vi "Add_Inlet_Temp_at_Z.vi"() -> (5 "Plug in titles":string[](array[string]), 7 "Plug in values":string[](array[string]))   [LabVIEW 2015]
uses:
  Globals/Meas_global.vi
panel:
  out "Z":dbl
  # "Please enter any run information in the box below"
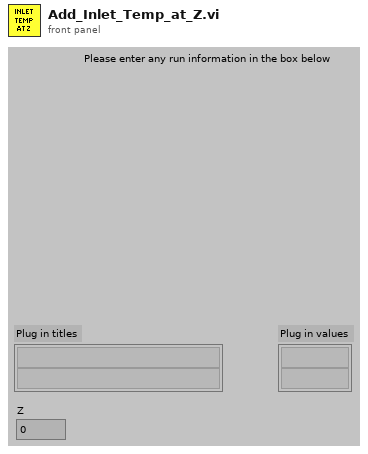
[diagram p1: front panel]
types:
  T1 = typedef "Analysis_info_cluster.ctl" = cluster{"Colour":u32, "Inst type":T2, "Inst name":string, "Symbol":string, "Code name":string, "Extra Info":string, "Inst Array":T3, "Extra Titles":string[], "Extra Values":string[], "U":dbl, "u^2":dbl, "u^3":dbl, "u^4":dbl, "Skew_u":dbl, "Kurt_u":dbl, "Sd Error in Mean":dbl, "% u'/U":dbl, "X":dbl, "Y":dbl, "Z":dbl, "Timescale integral to 25%":dbl, "Sd Error in Variance":dbl, "Calib File":path, "Calib Constants":dbl[], "Output Position":bool, "Full Stats":bool, "Av Sampling Rate":dbl, "Av No of Samples":dbl, "Total Meas Time (s)":dbl, "ADAM Ch Name":string}
  T2 = typedef "Inst_type.ctl" = enum16{"Propeller anemometer", "Raw voltage", "Pressure Transducer", "Pitot-static tube", "Preston tube", "Hot wire", "Cross wire 1", "Cross wire 2", "Generic Linear", "Generic Polynomial", "Generic BackPoly", "Fast FID", "Thermocouple", "Cold wire", "Pulsed Wire", "LDA Vel", "LDA Tran time", "LDA Arr time", "Microphone"}
  T3 = typedef "Instrument_Array.ctl" = enum16{"PWA", "LDA", "Analogue"}
  T4 = typedef "Post_Process.ctl" = enum16{"Take New Data", "Post Process Raw Data File"}
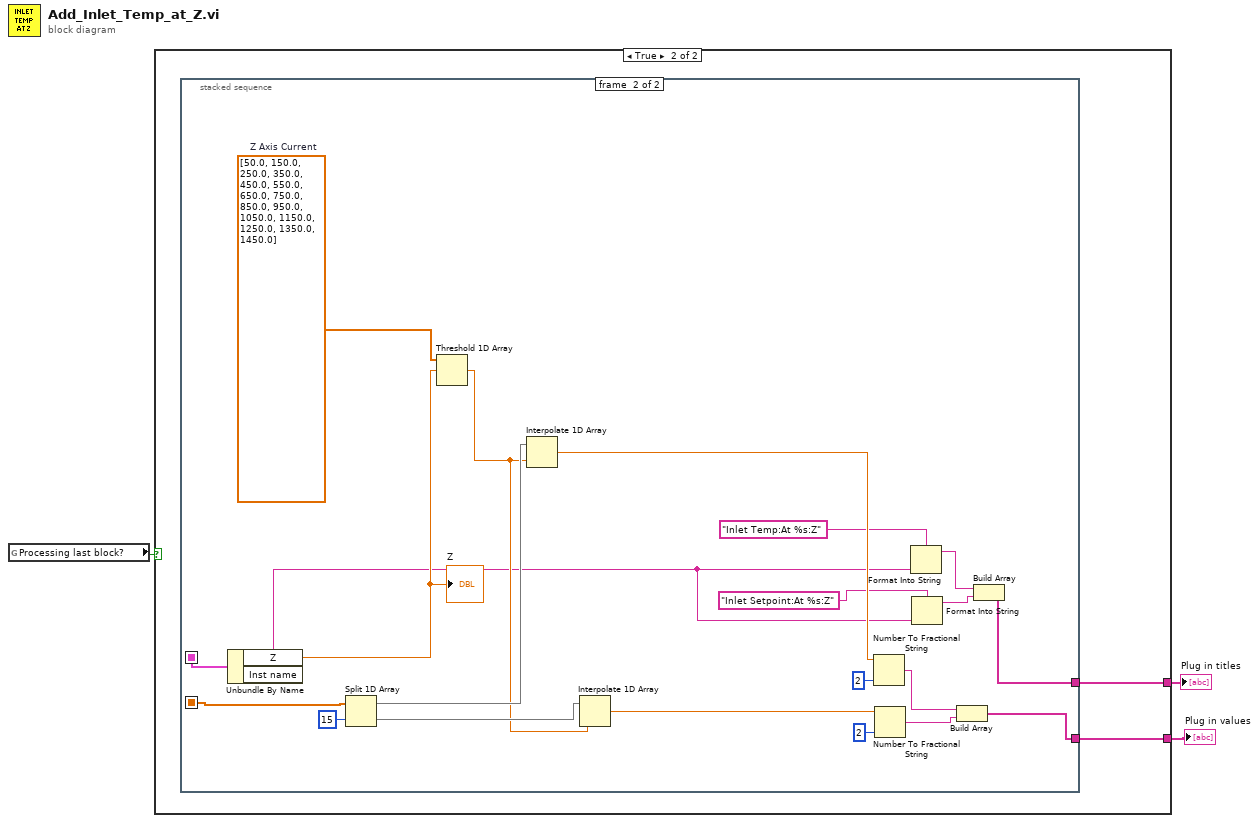
[diagram p0: block diagram]
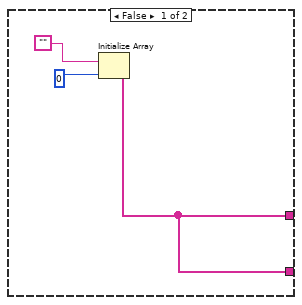
[diagram p2: hidden frame]
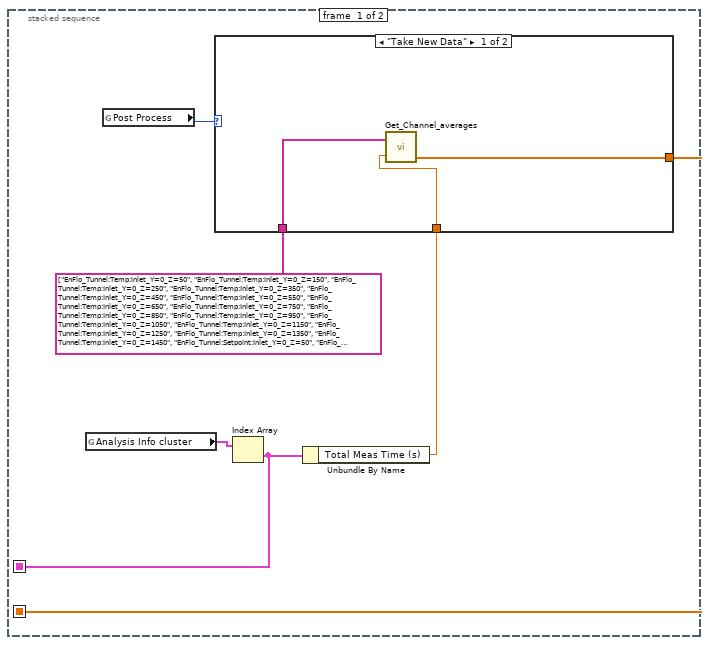
[diagram p3: hidden frame]
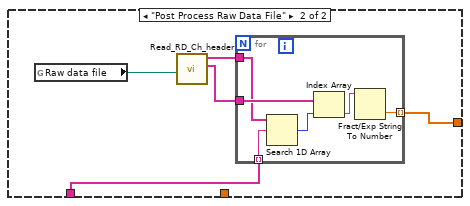
[diagram p4: hidden frame]
diagram:
  n1 = global read "Meas_global.vi" "Processing last block?"() -> (w3:bool)
  n2 = case shown="True" w3 {
    tunnel: [w4 w7] -> w2
    tunnel: [w4 w8] -> w1
    frame False {
      n3 = Initialize Array("", 0) -> (w4:string[])
    }
    frame True {
      n4 = stacked-sequence {
        seq-local: [w11 _] -> [_ w49]
        seq-local: [w9 _] -> [_ w40]
        tunnel: [_ w45] -> w8
        tunnel: [_ w44] -> w7
        frame #0 {
          n5 = global read "Meas_global.vi" "Analysis Info cluster"() -> (w12:T1[])
          n6 = global read "Meas_global.vi" "Post Process"() -> (w14:T4)
          n7 = Index Array(array=w12) -> (element=w11:T1)  [unwired: 1 in]
          n8 = Unbundle By Name(w11) -> ("Total Meas Time (s)"=w10:dbl)
          n9 = case shown="\"Take New Data\"" w14 {
            tunnel: string[] ["EnFlo_Tunnel:Temp:Inlet_Y=0_Z=50", "EnFlo_Tunnel:Temp:Inlet_Y=0_Z=150", "EnFlo_Tunnel:Temp:Inlet_Y=0_Z=250", "EnFlo_Tunnel:Temp:Inlet_Y=0_Z=350", "EnFlo_Tunnel:Temp:Inlet_Y=0_Z=450", "EnFlo_Tunnel:Temp:Inlet_Y=0_Z=550", "EnFlo_Tunnel:Temp:Inlet_Y=0_Z=650", "EnFlo_Tunnel:Temp:Inlet_Y=0_Z=750", "EnFlo_Tunnel:Temp:Inlet_Y=0_Z=850", "EnFlo_Tunnel:Temp:Inlet_Y=0_Z=950", "EnFlo_Tunnel:Temp:Inlet_Y=0_Z=1050", "EnFlo_Tunnel:Temp:Inlet_Y=0_Z=1150", "EnFlo_Tunnel:Temp:Inlet_Y=0_Z=1250", "EnFlo_Tunnel:Temp:Inlet_Y=0_Z=1350", "EnFlo_Tunnel:Temp:Inlet_Y=0_Z=1450", "EnFlo_Tunnel:Setpoint:Inlet_Y=0_Z=50", "EnFlo_Tunnel:Setpoint:Inlet_Y=0_Z=150", "EnFlo_Tunnel:Setpoint:Inlet_Y=0_Z=250", "EnFlo_Tunnel:Setpoint:Inlet_Y=0_Z=350", "EnFlo_Tunnel:Setpoint:Inlet_Y=0_Z=450", "EnFlo_Tunnel:Setpoint:Inlet_Y=0_Z=550", "EnFlo_Tunnel:Setpoint:Inlet_Y=0_Z=650", "EnFlo_Tunnel:Setpoint:Inlet_Y=0_Z=750", "EnFlo_Tunnel:Setpoint:Inlet_Y=0_Z=850", "EnFlo_Tunnel:Setpoint:Inlet_Y=0_Z=950", "EnFlo_Tunnel:Setpoint:Inlet_Y=0_Z=1050", "EnFlo_Tunnel:Setpoint:Inlet_Y=0_Z=1150", "EnFlo_Tunnel:Setpoint:Inlet_Y=0_Z=1250", "EnFlo_Tunnel:Setpoint:Inlet_Y=0_Z=1350", "EnFlo_Tunnel:Setpoint:Inlet_Y=0_Z=1450"] ("Sub set") -> [w17 w19]
            tunnel: [w16 w18] -> w9
            tunnel: w10 -> [w15 _]
            frame "Take New Data" {
              n10 = call "Get_Channel_averages.vi"("Desired Ch Names"=w17, "Averaging time (mins)"=w15) -> ("number"=w16:dbl[])  [unwired: 1 in, 2 out]
            }
            frame "Post Process Raw Data File" {
              n11 = global read "Meas_global.vi" "Raw data file"() -> (w22:path)
              n12 = call "Read_RD_Ch_header.vi"("Raw data file"=w22) -> ("Ch Name Out"=w20:string[], "Ch Values"=w21:string[])  [unwired: 2 out]
              n13 = for {
                tunnel: w21 -> [w28]
                tunnel: w20 -> [w27]
                tunnel: w19 -> [w26] mode=indexing
                tunnel: [w23] -> w18 mode=indexing
                n14 = Search 1D Array(1D array=w27, element=w26) -> (index of element=w25:i32)  [unwired: 1 in]
                n15 = Index Array(array=w28, index=w25) -> (element=w24:string)
                n16 = Fract/Exp String To Number(string=w24) -> (number=w23:dbl)  [unwired: 3 in, 1 out]
              }
            }
          }
        }
        frame #1 {
          w48 = dbl[] [50.0, 150.0, 250.0, 350.0, 450.0, 550.0, 650.0, 750.0, 850.0, 950.0, 1050.0, 1150.0, 1250.0, 1350.0, 1450.0]  # Z Axis Current
          n17 = Unbundle By Name(w49) -> ("Z"=w47:dbl, "Inst name"=w33:string)
          "Z" <- w47
          n18 = Split 1D Array(array=w40, index=15) -> (first subarray=w38:dbl[], second subarray=w37:dbl[])
          n19 = Threshold 1D Array(2:w47, 3:w48) -> (0:w36:dbl)  [unwired: 1 in]
          n20 = Interpolate 1D Array(1:w36, 2:w38) -> (0:w46:dbl)
          n21 = Interpolate 1D Array(1:w36, 2:w37) -> (0:w29:dbl)
          n22 = Number To Fractional String(number=w46, precision (6)=i16 2) -> (F-format string=w35:string)  [unwired: 2 in]
          n23 = Number To Fractional String(number=w29, precision (6)=i16 2) -> (F-format string=w30:string)  [unwired: 2 in]
          n24 = Format Into String(format string="Inlet Temp:At %s:Z", w33) -> (resulting string=w42:string)  [unwired: 2 in, 1 out]
          n25 = Format Into String(format string="Inlet Setpoint:At %s:Z", w33) -> (resulting string=w32:string)  [unwired: 2 in, 1 out]
          n26 = Build Array(w35, w30) -> (w45:string[])
          n27 = Build Array(w42, w32) -> (w44:string[])
        }
      }
    }
  }
  "Plug in titles" <- w2
  "Plug in values" <- w1
